vi "RadWag Tare Set And Read.vi"() -> ()   [LabVIEW 2016]
doc: "This VI tares the balance and reads tare value afterwards. Tare can be performed with current mass value or with one set by user."
uses:
  <instrlib>/RadWag balances and scales/RadWag balances and scales.lvlib
panel:
  out "Tare Unit":string
  out "Tare Value":dbl format="%#.6f"
  in  "Tare Value [g]":dbl
  in  "Set Value (F:Tare with current value)":bool
  in  "VISA resource name":refnum<visa-resource-name>
  # "(c) 2014 Przemysłowy Instytut Automatyki i Pomiarów PIAP.  ALL RIGHTS RESERVED."
  # "Set tare source and value\n before running this VI."
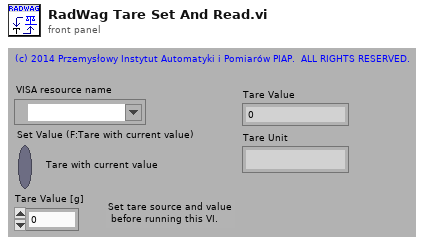
[diagram p1: front panel]
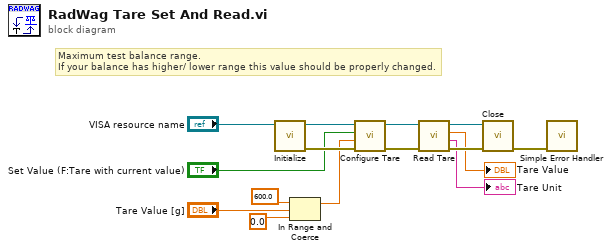
[diagram p0: block diagram]
diagram:
  # "Maximum test balance range.\nIf your balance has higher/ lower range this value should be properly changed."
  n1 = call <instrlib>:"Initialize.vi"("VISA resource name"="VISA resource name") -> ("error out"=w14:errorcluster, "VISA resource name out"=w15:refnum<visa-resource-name>)  [unwired: 9 in]
  n2 = In Range and Coerce(upper limit=600.0, x="Tare Value [g]", lower limit=0.0) -> (coerced(x)=w5:dbl)  [unwired: 1 out]
  n3 = call <instrlib>:"Configure Tare.vi"("error in (no error)"=w14, "Tare Value [g]"=w5, "Set Value (F:Tare with current value)"="Set Value (F:Tare with current value)", "VISA resource name"=w15) -> ("error out"=w11:errorcluster, "VISA resource name out"=w12:refnum<visa-resource-name>)  [unwired: 6 in]
  n4 = call <instrlib>:"Read Tare.vi"("error in (no error)"=w11, "VISA resource name"=w12) -> ("error out"=w3:errorcluster, "Tare Unit"=→"Tare Unit":string, "Tare Value"=→"Tare Value":dbl, "VISA resource name out"=w4:refnum<visa-resource-name>)  [unwired: 6 in]
  n5 = call <instrlib>:"Close.vi"("error in (no error)"=w3, "VISA resource name"=w4) -> ("error out"=w13:errorcluster)  [unwired: 9 in]
  n6 = call <vilib>:"Simple Error Handler.vi"("error in (no error)"=w13) -> ()  [unwired: 4 in, 5 out]
